vi "Start Call (Command).vi"(6 "Event References":T1, 7 "Configuration":refnum<class "configuration.lvclass">, 8 "error in":errorcluster, 9 "Working Directory (default <Not A Path> - System Default)":path=path "" caption="Working Directory", 11 "Command":string) -> (0 "error out":errorcluster, 3 "New ASE Handle":refnum<class "ase.lvclass">)   [LabVIEW 2024, in "serenial.io-ase.lvlib" / "ase.lvclass"]
doc: "<B>Start an Asynchronous System Executable Call</B>\n\nThe command input should contain the executable name (which will be found using the System's Path Environmental Variable) and any arguments that should be supplied. See the \"examples of the cmd style calls\" from the boost documentation at https://www.boost.org/doc/libs/1_77_0/doc/html/boost_process/design.html#boost_process.design.arg_cmd_style.\n\nThe User Events References to generate the \"Did Launch\", \"Standard Output\", \"Standard Error\" and \"Did Exit\" events can be supplied or omitted as required. <B>Ensure that the event registration process for any User Events passed to this VI has already been undertaken</B>.\n\nThe configuration class allows for override of certain behaviours such as the regular expression used to match the breaks in the Standard Out and Standard Error to be specified.\n\nThis VI generates the following errors:\n-4601: Poorly formatted/incorrect Regular Expression supplied.\n-5691000: Internal Library Error. <Check Error Message for more details>\n-5691301: Unable to launch the executable. <Check Error Message for more details>\n-5691305: Executable paths parameter cannot be an empty value."
uses:
  ase.lvclass
  Event References.ctl
  Standard Output.ctl
  Standard Error.ctl
  Did Exit.ctl
  configuration/configuration.lvclass
  ase.lvclass/ase.ctl
  Error Empty Executable Name.vi
  Check Shared Library Version.vi
  Merge Call Library Errors.vi
  Trim Whitespace.vi
  Error Internal Library Implementation Error.vi
  <vilib>/Utility/error.llb/Error Cluster From Error Code.vi
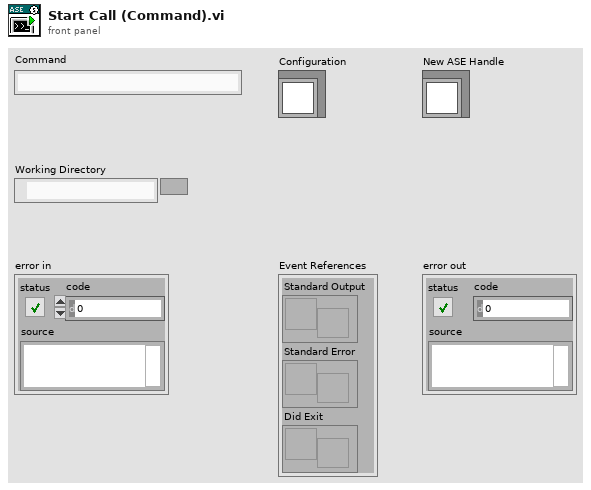
[diagram p1: front panel]
types:
  T1 = typedef "serenial.io-ase.lvlib/ase.lvclass/Event References.ctl" = cluster{"Standard Output":refnum<user-event>, "Standard Error":refnum<user-event>, "Did Exit":refnum<user-event>}
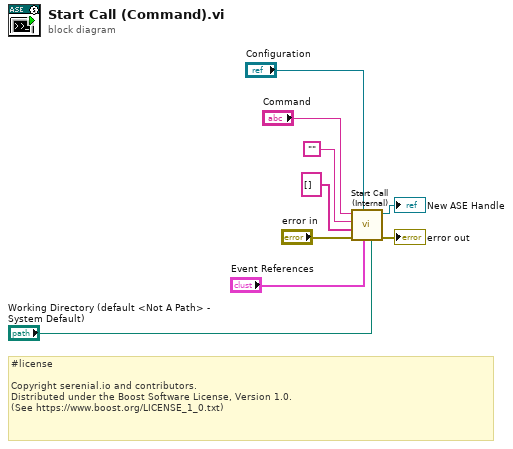
[diagram p0: block diagram]
diagram:
  # "#license\n\nCopyright serenial.io and contributors.\nDistributed under the Boost Software License, Version 1.0.\n(See https://www.boost.org/LICENSE_1_0.txt)"
  n1 = call "Start Call (Internal).vi"("Working Directory (default <Not A Path> - System Default)"="Working Directory (default <Not A Path> - System Default)", "Event References"="Event References", "Configuration"="Configuration", "error in"="error in", "Arguments"=string[] [], "Exe"="", "Command"="Command") -> ("error out"=→"error out":errorcluster, "New ASE Handle"=→"New ASE Handle":refnum<class "ase.lvclass">)  [unwired: 3 in]
